vi "compatWriteText.vi"(5 "convert eol (F)":bool, 6 "data":string, 7 "header (F)":bool, 8 "error in":errorcluster, 11 "refnum":refnum<file>) -> (0 "error out":errorcluster, 3 "dup refnum":refnum<file>)   [LabVIEW 2020]
doc: "Compatibility VI to preserve the functionality of the LabVIEW 7.1 Write File primitive."
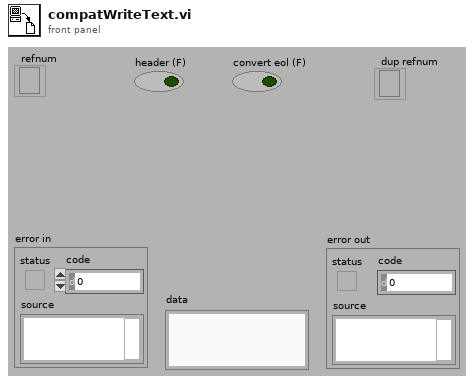
[diagram p1: front panel]
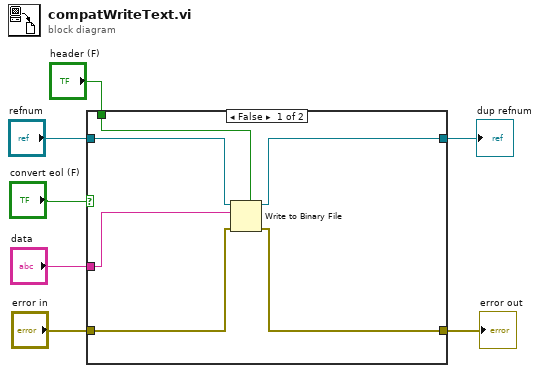
[diagram p0: block diagram]
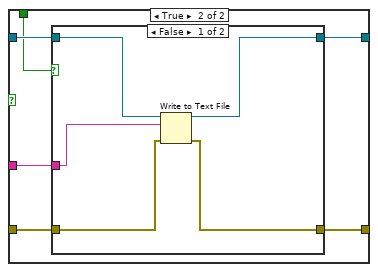
[diagram p2: hidden frame]
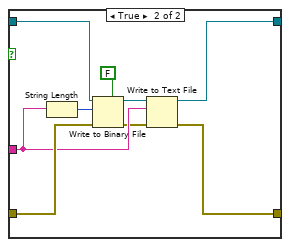
[diagram p3: hidden frame]
diagram:
  n1 = case shown="False" "convert eol (F)" {
    tunnel: "header (F)" -> [w8 w15]
    tunnel: "refnum" -> [w13 w17]
    tunnel: "error in" -> [w12 w19]
    tunnel: [w11 w18] -> w3
    tunnel: [w10 w16] -> w2
    tunnel: "data" -> [w9 w14]
    frame False {
      n2 = Write to Binary File(file (use dialog)=w13, data=w9, error in=w12, 5:w8) -> (refnum out=w10:refnum<file>, error out=w11:errorcluster)  [unwired: 2 in, 1 out]
    }
    frame True {
      n3 = case shown="False" w15 {
        tunnel: w19 -> [w23 w33]
        tunnel: [w22 w32] -> w18
        tunnel: w17 -> [w21 w30]
        tunnel: [w20 w31] -> w16
        tunnel: w14 -> [w24 w29]
        frame False {
          n4 = Write to Text File(file (use dialog)=w21, text=w24, error in=w23) -> (refnum out=w20:refnum<file>, error out=w22:errorcluster)  [unwired: 1 in, 1 out]
        }
        frame True {
          n5 = String Length(string=w29) -> (length=w25:i32)
          n6 = Write to Binary File(file (use dialog)=w30, data=w25, error in=w33, 5:FALSE ("prepend array or string size? (T)")) -> (refnum out=w28:refnum<file>, error out=w27:errorcluster)  [unwired: 2 in, 1 out]
          n7 = Write to Text File(file (use dialog)=w28, text=w29, error in=w27) -> (refnum out=w31:refnum<file>, error out=w32:errorcluster)  [unwired: 1 in, 1 out]
        }
      }
    }
  }
  "dup refnum" <- w2
  "error out" <- w3
